vi "NewTweet.vi"(11 "Message Main Body":string="Error occurred") -> ()   [LabVIEW 2013]
doc: "This example posts a text only tweet."
uses:
  <vilib>/LVH/i3 OAuth/Controls/Credentials.ctl
  <vilib>/LVH/i3 Twitter/SubVIs/Twitter Open - Desktop.vi
  <vilib>/LVH/i3 Twitter/Tweets/Post Tweet.vi
  <vilib>/LVH/i3 Twitter/i3-twitter.lvlib
  <vilib>/LVH/i3 OAuth/i3-oauth.lvlib
panel:
  in  "Consumer Secret":string="OLVXP1iuy8bhR5U5btmpMGRuPD8rVhVQv722w70INby6Mns2pd"
  in  "Consumer Key":string="xIcnxFzcuRh07kReATPijMtuV"
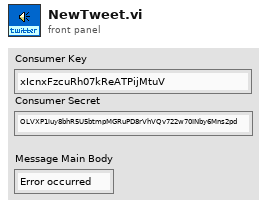
[diagram p1: front panel]
types:
  T1 = typedef "i3-oauth.lvlib/Credentials.ctl" = cluster{"Token":string, "Secret":string}
  T2 = typedef "i3-twitter.lvlib/Twitter Handle.ctl" = cluster{"OAuth Credentials":T3, "since ID":string, "max ID":string, "Screen Name":string}
  T3 = typedef "i3-oauth.lvlib/OAuth Handle.ctl" = cluster{"Signature Method":T4, "Version":string, "Client":T1, "Access":T1}
  T4 = typedef "i3-oauth.lvlib/Signature Method.ctl" = enum16{"HMAC-MD5", "HMAC-SHA1", "HMAC-SHA224", "HMAC-SHA256", "HMAC-SHA384", "HMAC-SHA512"}
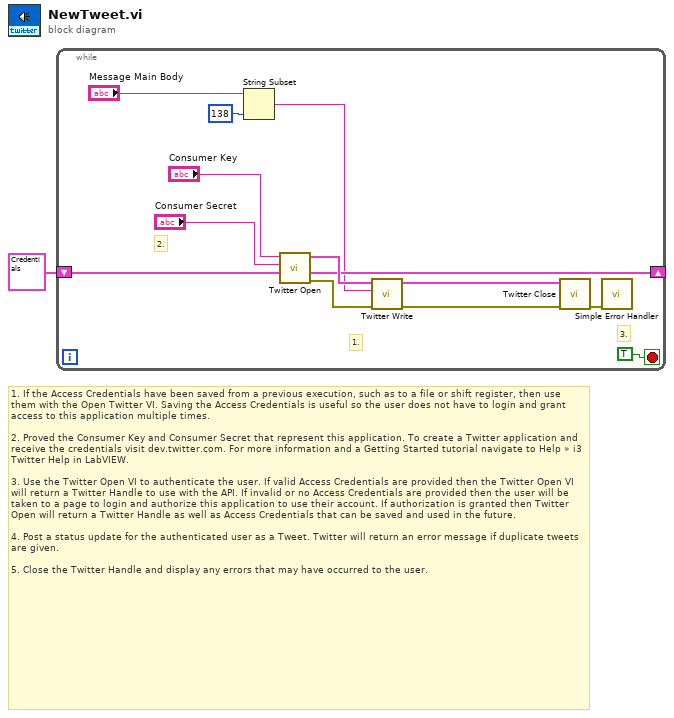
[diagram p0: block diagram]
diagram:
  # "1. If the Access Credentials have been saved from a previous execution, such as to a file or shift register, then use them with the Open Twitter VI. Saving the Access Credentials is useful so the user does not have to login and grant access to this application multiple times.\n\n2. Proved the Consumer Key and Consumer Secret that represent this application. To create a Twitter application and receive the credentials visit dev.twitter.com. For more information and a Getting Started tutorial navigate to Help » i3 Twitter Help in LabVIEW.\n\n3. Use the Twitter Open VI to authenticate the user. If valid Access Credentials are provided then the Twitter Open VI will return a Twitter Handle to use with the API. If invalid or no Access Credentials are provided then the user will be taken to a page to login and authorize this application to use their account. If authorization is granted then Twitter Open will return a Twitter Handle as well as Access Credentials that can be saved and used in the future.\n\n4. Post a status update for the authenticated user as a Tweet. Twitter will return an error message if duplicate tweets are given.\n\n5. Close the Twitter Handle and display any errors that may have occurred to the user."
  n1 = while {
    shift-right: [w10] -> _
    shift-left: T1 {"Token"="2615910943-vJw5MPX2QthQbdi03GvsIzeeCfAB0FfIzSPfJiy", "Secret"="YGywkYXe6O198k6OxPvGjegudxKvuk8gGQpfOHJDnamdq"} ("Access Credentials (out)") -> [w7]
    stop <- TRUE stop-if-true
    # "3."
    # "2."
    # "1."
    n2 = String Subset(string="Message Main Body", length (rest)=138 ("length (rest)")) -> (substring=w5:string)  [unwired: 1 in]
    n3 = call-poly <vilib>:"Twitter Open.vi"("Access Credentials (in)"=w7, "Consumer Secret"="Consumer Secret", "Consumer Key"="Consumer Key") -> ("error out"=w14:errorcluster, "Access Credentials (out)"=w10:T1, "Twitter Handle Out"=w13:T2)  [unwired: 6 in]
    n4 = call-poly <vilib>:"Twitter Write.vi"("error in (no error)"=w14, "Tweet"=w5, "Twitter Handle In"=w13) -> ("error out"=w3:errorcluster, "Twitter Handle Out"=w2:T2)  [unwired: 7 in]
    n5 = call <vilib>:"Twitter Close.vi"("error in"=w3, "Twitter Handle In"=w2) -> ("error out"=w8:errorcluster)  [unwired: 9 in]
    n6 = call <vilib>:"Simple Error Handler.vi"("error in (no error)"=w8) -> ()  [unwired: 4 in, 5 out]
  }
